vi "Connect.vi"   [LabVIEW 2017, in "LabSFTP.lvlib"]
doc: "<License>This software is distributed under the BSD 3-Clause License. For the full license please see license.txt or visit www.labvolution.com/license</License>"
uses:
  LabSFTP.lvlib
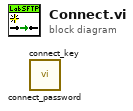
[diagram p0: block diagram]
diagram:
  n1 = call "connect_password.vi"() -> ()  [unwired: 9 in, 3 out]
  n2 = call "connect_key.vi"() -> ()  [unwired: 9 in, 3 out]
